vi "Dialog.vi"(10 "Name":string) -> (1 "Name 2":string)   [LabVIEW 2017]
panel:
  out "OK-Schaltfläche 3":bool
  in  "OK-Schaltfläche 2":bool
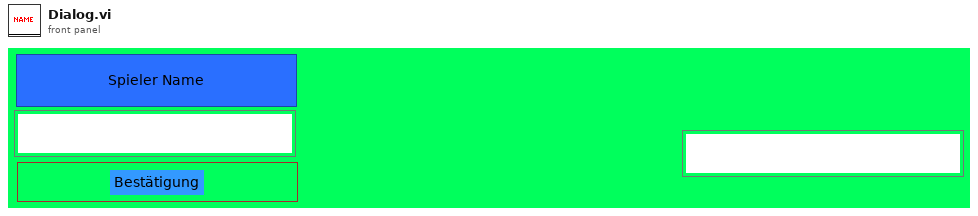
[diagram p1: front panel]
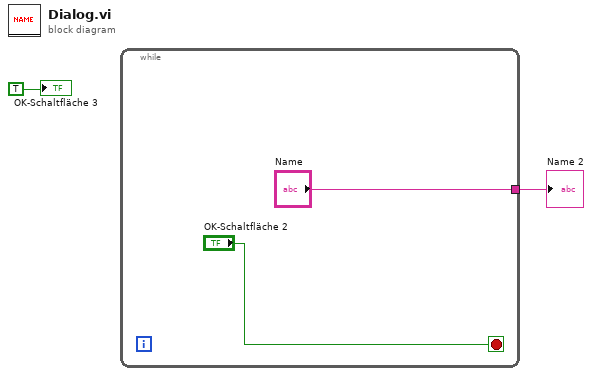
[diagram p0: block diagram]
diagram:
  n1 = while {
    tunnel: ["Name"] -> w2
    stop <- "OK-Schaltfläche 2" stop-if-true
  }
  "Name 2" <- w2
  "OK-Schaltfläche 3" <- TRUE
